vi "api_DeleteDVR.vi"(8 "error in (no error)":errorcluster, 11 "data value reference":refnum<data-value>) -> (0 "error out":errorcluster)   [LabVIEW 2019, in "ConfigClass.lvlib" / "ConfigClass.lvclass"]
uses:
  ConfigClass.lvclass
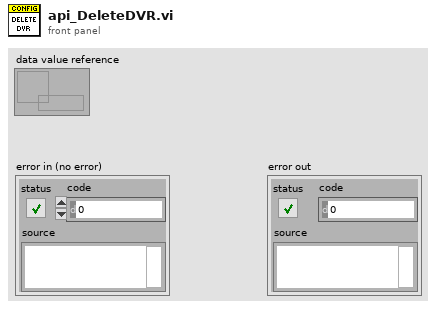
[diagram p1: front panel]
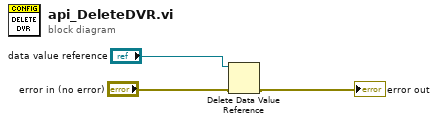
[diagram p0: block diagram]
diagram:
  n1 = Delete Data Value Reference(data value reference="data value reference", error in="error in (no error)") -> (error out=→"error out":errorcluster)  [unwired: 1 out]
